vi "PotRead.vi"(0 "PotDevRef":T1={"DevStatus"={"status"=FALSE, "code"=0, "source"=""}, "Analog Channel"=enum."Invalid"}, 1 "Pot_Filter_Percent":dbl=0.8, 2 "mV/deg":dbl=1.389 format="%#_13g", 3 "upper limit":dbl=3300.0, 4 "lower limit":dbl=300.0) -> (5 "In_Range?":bool, 6 "Pot":dbl)   [LabVIEW 2016]
uses:
  <vilib>/Rock Robotics/WPI/AnalogChannel/WPI_AnalogChannelDevRef.ctl
  <vilib>/Rock Robotics/SystemInterfaces/AI/FPGA_AIChannel.ctl
panel:
  out "Waveform Chart":cluster{dbl, "Out":dbl}(graph)
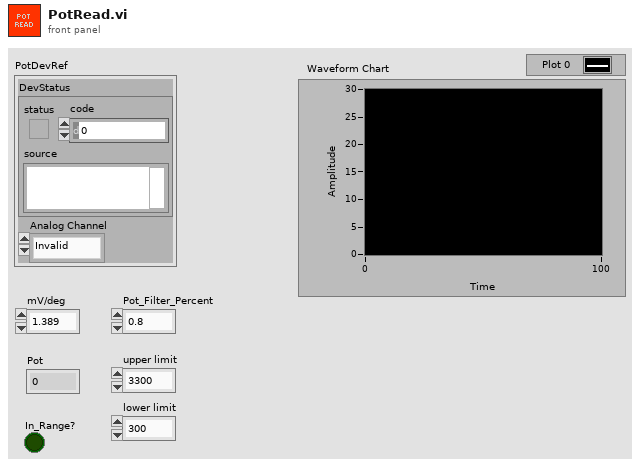
[diagram p1: front panel]
types:
  T1 = typedef "WPI_AnalogChannelDevRef.ctl" = cluster{"DevStatus":errorcluster, "Analog Channel":T2}
  T2 = typedef "FPGA_AIChannel.ctl" = enum8{"AI 0", "AI 1", "AI 2", "AI 3", "AI MXP 0", "AI MXP 1", "AI MXP 2", "AI MXP 3", "Invalid"}
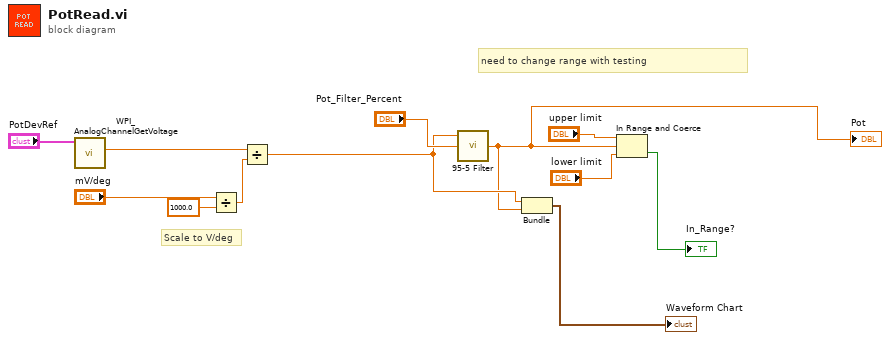
[diagram p0: block diagram]
diagram:
  # "Scale to V/deg"
  # "need to change range with testing"
  n1 = call <vilib>:"WPI_AnalogChannelGetVoltage.vi"("AIDeviceRef"="PotDevRef") -> ("Voltage"=w12:dbl)  [unwired: 8 in, 2 out]
  n2 = Divide(x="mV/deg", y=1000.0) -> (x/y=w3:dbl)
  n3 = Divide(x=w12, y=w3) -> (x/y=w8:dbl)
  n4 = call "95-5 Filter.vi"("Percent"="Pot_Filter_Percent", "In"=w8) -> ("Out"=w7:dbl)  [unwired: 1 in]
  "Pot" <- w7
  n5 = Bundle(w8, "Out"=w7) -> (→"Waveform Chart":cluster{dbl, "Out":dbl})  [unwired: 1 in]
  n6 = In Range and Coerce(upper limit="upper limit", x=w7, lower limit="lower limit") -> (In Range?=→"In_Range?":bool)  [unwired: 1 out]
